vi "Decode.vi"(8 "error in (no error)":errorcluster, 10 "Binary string in":string, 11 "obj in":refnum<class "Pupil.lvclass">) -> (0 "error out":errorcluster, 1 "Data out":refnum<class "Data.lvclass">, 2 "Rest of binary string":string, 3 "obj out":refnum<class "Pupil.lvclass">)   [LabVIEW 2020, in "Pupil.lvclass"]
uses:
  Pupil.lvclass
  Data Class/Data.lvclass
  Data Class/Datatypes/Data_Pupil_class/Attribute.vi
  Pupil.lvclass/Pupil.ctl
  Data Class/Datatypes/Data_Pupil_class/Data_Pupil.lvclass
  C:/Users/theod/Desktop/API - EyeT data streaming to IC/Smart Eye API/Source/Classes/Smart Eye Pro Drivers/Data Class/Data.lvclass
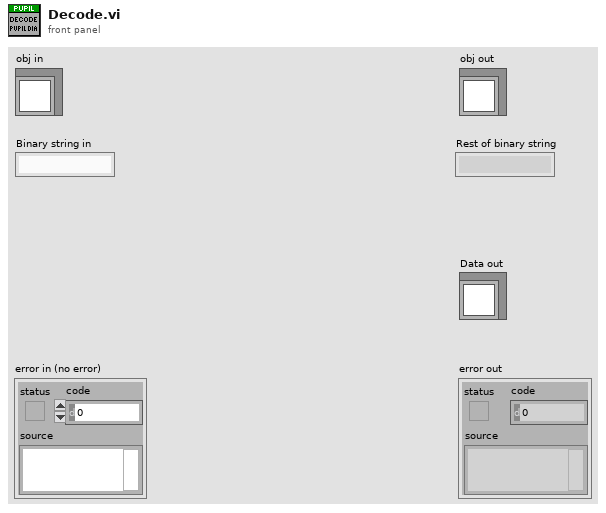
[diagram p1: front panel]
types:
  T1 = typedef "Data_Pupil.lvclass/Attribute.vi" = cluster{"PupilDiameter":dbl, "LeftPupilDiameter":dbl, "LeftPupilDiameterQ":dbl, "RightPupilDiameter":dbl, "RightPupilDiameterQ":dbl}
  T2 = enum16{"big-endian, network order", "native, host order", "little-endian"}
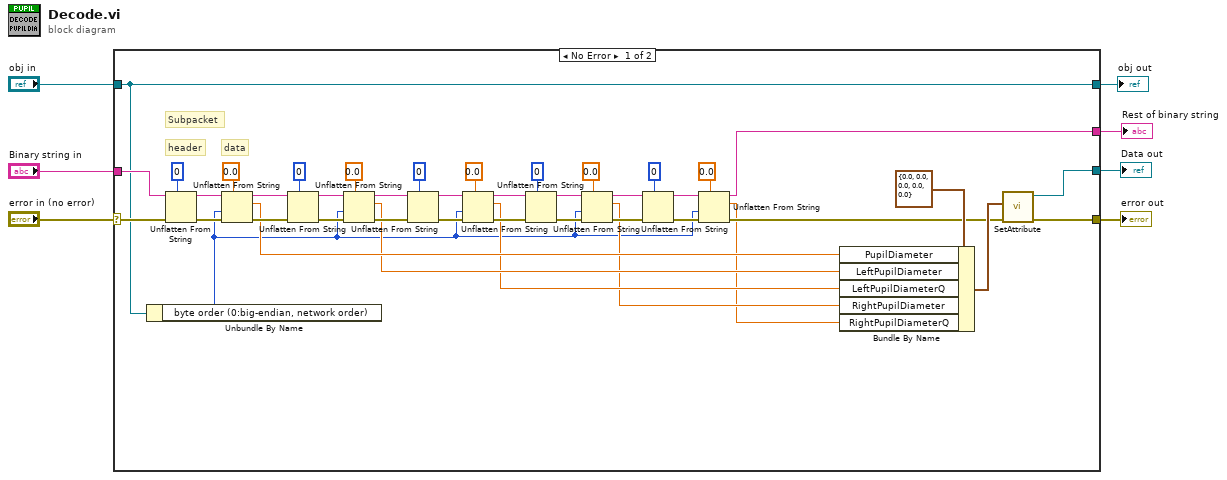
[diagram p0: block diagram]
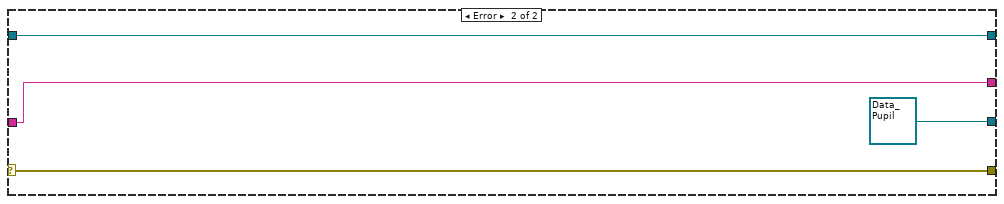
[diagram p2: hidden frame]
diagram:
  n1 = case shown="No Error" "error in (no error)" {
    selector: "error in (no error)" -> [w18 w52]
    tunnel: [w48 w52] -> w6
    tunnel: "obj in" -> [w9 w51]
    tunnel: [w9 w51] -> w4
    tunnel: "Binary string in" -> [w11 w49]
    tunnel: [w45 refnum<class "Data_Pupil.lvclass"> refnum ("Data_Pupil_Diameter")] -> w2
    tunnel: [w10 w49] -> w1
    frame No Error {
      # "header"
      # "data"
      # "Subpacket"
      n2 = Unbundle By Name(w9) -> ("byte order (0:big-endian, network order)"=w8:T2)
      n3 = Unflatten From String(type=u32 0, binary string=w11, error in (no error)=w18) -> (rest of the binary string=w42:string, error out=w33:errorcluster)  [unwired: 2 in, 1 out]
      n4 = Unflatten From String(type=0.0, binary string=w42, byte order (0:big-endian, network order)=w8, error in (no error)=w33) -> (rest of the binary string=w41:string, value=w16:dbl, error out=w31:errorcluster)  [unwired: 1 in]
      n5 = Unflatten From String(type=u32 0, binary string=w41, error in (no error)=w31) -> (rest of the binary string=w43:string, error out=w32:errorcluster)  [unwired: 2 in, 1 out]
      n6 = Unflatten From String(type=0.0, binary string=w43, byte order (0:big-endian, network order)=w8, error in (no error)=w32) -> (rest of the binary string=w44:string, value=w15:dbl, error out=w30:errorcluster)  [unwired: 1 in]
      n7 = Unflatten From String(type=0, binary string=w44) -> (rest of the binary string=w28:string)  [unwired: 3 in, 2 out]
      n8 = Unflatten From String(type=0.0, binary string=w28, byte order (0:big-endian, network order)=w8) -> (rest of the binary string=w26:string, value=w14:dbl)  [unwired: 2 in, 1 out]
      n9 = Unflatten From String(type=u32 0, binary string=w26, error in (no error)=w30) -> (rest of the binary string=w40:string, error out=w29:errorcluster)  [unwired: 2 in, 1 out]
      n10 = Unflatten From String(type=0.0, binary string=w40, byte order (0:big-endian, network order)=w8, error in (no error)=w29) -> (rest of the binary string=w21:string, value=w13:dbl, error out=w19:errorcluster)  [unwired: 1 in]
      n11 = Unflatten From String(type=u32 0, binary string=w21, error in (no error)=w19) -> (rest of the binary string=w25:string, error out=w22:errorcluster)  [unwired: 2 in, 1 out]
      n12 = Unflatten From String(type=0.0, binary string=w25, byte order (0:big-endian, network order)=w8, error in (no error)=w22) -> (rest of the binary string=w10:string, value=w12:dbl, error out=w17:errorcluster)  [unwired: 1 in]
      n13 = Bundle By Name(cluster=T1 {"PupilDiameter"=0.0, "LeftPupilDiameter"=0.0, "LeftPupilDiameterQ"=0.0, "RightPupilDiameter"=0.0, "RightPupilDiameterQ"=0.0} ("Set Attribute"), "PupilDiameter"=w16, "LeftPupilDiameter"=w15, "LeftPupilDiameterQ"=w14, "RightPupilDiameter"=w13, "RightPupilDiameterQ"=w12) -> (w46:T1)
      n14 = call "SetAttribute.vi"("error in (no error)"=w17, "Set Attribute"=w46) -> ("error out"=w48:errorcluster, "Data_Pupil_Diameter out"=w45:refnum<class "Data_Pupil.lvclass">)  [unwired: 8 in]
    }
    frame Error {
    }
  }
  "error out" <- w6
  "obj out" <- w4
  "Data out" <- w2
  "Rest of binary string" <- w1
